vi "FlatToRichnixnet_grpc_ConvertTimestamp1nsTo100nsRequest.vi"(5 "OutputClusterType":T1, 11 "InputCluster":T2) -> (3 "OutputCluster":T1)   [LabVIEW 2025, in "xnet-grpc_client.lvlib"]
uses:
  nixnet_grpc_ConvertTimestamp1nsTo100nsRequest_Flat.ctl
  nixnet_grpc_ConvertTimestamp1nsTo100nsRequest.ctl
  xnet-grpc_client.lvlib
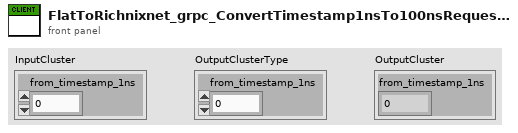
[diagram p1: front panel]
types:
  T1 = typedef "xnet-grpc_client.lvlib/nixnet_grpc_ConvertTimestamp1nsTo100nsRequest.ctl" = cluster{"from_timestamp_1ns":u64}
  T2 = typedef "xnet-grpc_client.lvlib/nixnet_grpc_ConvertTimestamp1nsTo100nsRequest_Flat.ctl" = cluster{"from_timestamp_1ns":u64}
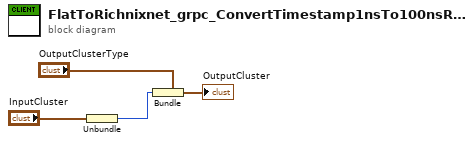
[diagram p0: block diagram]
diagram:
  n1 = Unbundle "Unbundle"("InputCluster") -> ("from_timestamp_1ns"=w1:u64)
  n2 = Bundle "Bundle"(cluster="OutputClusterType", "from_timestamp_1ns"=w1) -> (→"OutputCluster":T1)
